vi "PushElement.vi"(8 "error in (no error)":errorcluster, 10 "open list element":T1, 11 "Astar Open List in":refnum<class "NI_Robotics_Priority Queue.lvclass">) -> (0 "error out":errorcluster, 3 "Astar Open List out":refnum<class "NI_Robotics_Priority Queue.lvclass">)   [LabVIEW 2017, in "NI_Robotics_Priority Queue.lvclass"]
uses:
  <vilib>/robotics/Navigation/shared/Priority Queue/NI_Robotics_Priority Queue.lvclass
  <vilib>/robotics/Navigation/shared/Priority Queue/Open List Element.ctl
  <vilib>/robotics/Navigation/shared/MapNode/AbstractMapNode/NI_Robotics_AbstractMapNode.lvclass
  <vilib>/robotics/Navigation/shared/Priority Queue/NI_Robotics_Priority Queue.lvclass/NI_Robotics_Priority Queue.ctl
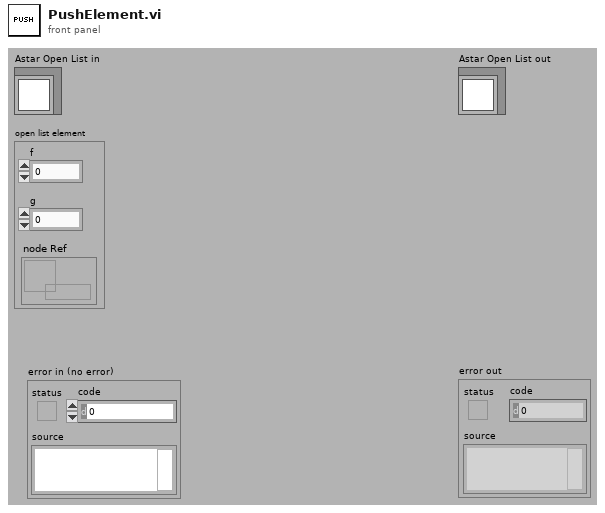
[diagram p1: front panel]
types:
  T1 = typedef "NI_Robotics_Priority Queue.lvclass/Open List Element.ctl" = cluster{"f":dbl, "g":dbl, "node Ref":refnum<data-value>}
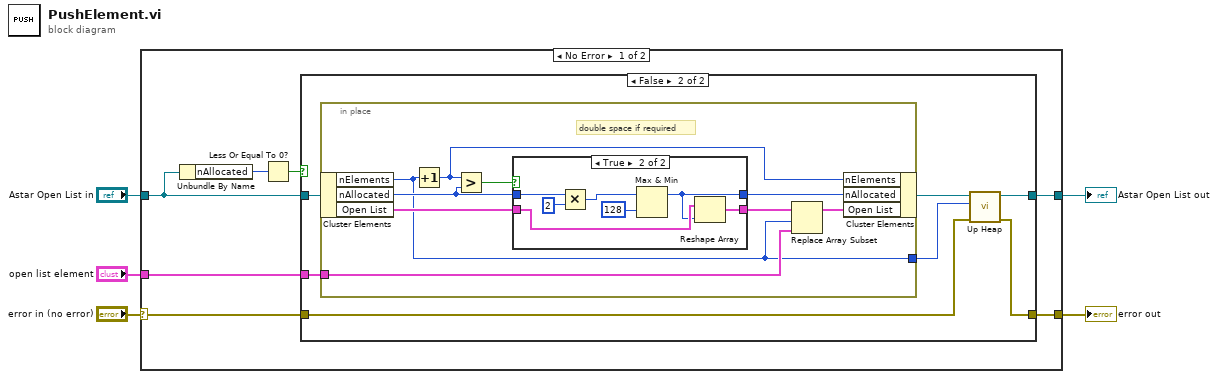
[diagram p0: block diagram]
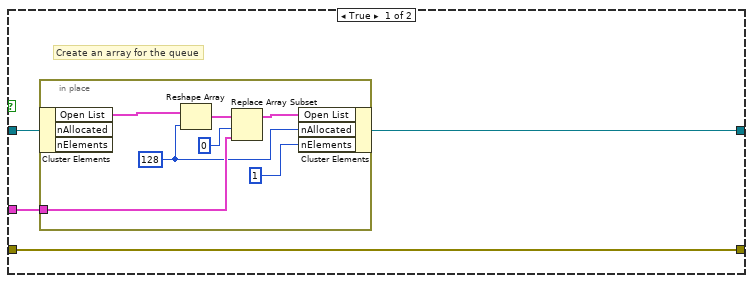
[diagram p2: hidden frame]
diagram:
  n1 = case shown="No Error" "error in (no error)" {
    selector: "error in (no error)" -> [w6 w49]
    tunnel: "Astar Open List in" -> [w12 w50]
    tunnel: "open list element" -> [w11 _]
    tunnel: [w10 w50] -> w3
    tunnel: [w9 w49] -> w2
    frame No Error {
      n2 = Unbundle By Name(w12) -> ("nAllocated"=w8:i32)
      n3 = Less Or Equal To 0?(x=w8) -> (x <= 0?=w7:bool)
      n4 = case shown="False" w7 {
        tunnel: w12 -> [w16 w30]
        tunnel: w11 -> [w15 w29]
        tunnel: [w14 w26] -> w10
        tunnel: w6 -> [w13 w25]
        tunnel: [w13 w24] -> w9
        frame True {
          # "Create an array for the queue"
          n5 = in-place {
            in-place-border: w15 -> [w20]
            w19 = 128 ("dimension size")
            n6 = in-place-cluster #1(w16) -> ("Open List"=w23:T1[])  [unwired: 2 out]
            n7 = Reshape Array(w23, w19) -> (w22:T1[])
            n8 = Replace Array Subset(array=w22, new element=w20, index=0) -> (w18:T1[])
            n9 = in-place-cluster #1("Open List"=w18, "nAllocated"=w19, "nElements"=1) -> (w14:refnum<class "NI_Robotics_Priority Queue.lvclass">)
          }
        }
        frame False {
          n10 = in-place {
            in-place-border: w29 -> [w34]
            in-place-border: [w31] -> w28
            # "double space if required"
            n11 = in-place-cluster #2(w30) -> ("nElements"=w31:i32, "nAllocated"=w38:i32, "Open List"=w37:T1[])
            n12 = Increment(x=w31) -> (x+1=w33:i32)
            n13 = Greater?(x=w33, y=w38) -> (0:w39:bool)
            n14 = case shown="True" w39 {
              tunnel: w38 -> [w41 w48]
              tunnel: w37 -> [w40 w44]
              tunnel: [w40 w43] -> w35
              tunnel: [w41 w42] -> w36
              frame False {
              }
              frame True {
                n15 = Multiply(x=w48, y=2) -> (x*y=w46:i32)
                n16 = Max & Min(x=w46, y=128) -> (max(x,y)=w42:i32)  [unwired: 1 out]
                n17 = Reshape Array(w44, w42) -> (w43:T1[])
              }
            }
            n18 = Replace Array Subset(array=w35, new element=w34, index=w31) -> (w32:T1[])
            n19 = in-place-cluster #2("nElements"=w33, "nAllocated"=w36, "Open List"=w32) -> (w27:refnum<class "NI_Robotics_Priority Queue.lvclass">)
          }
          n20 = call <vilib>:"Up Heap.vi"("error in (no error)"=w25, "index"=w28, "Astar Open List in"=w27) -> ("error out"=w24:errorcluster, "Astar Open List out"=w26:refnum<class "NI_Robotics_Priority Queue.lvclass">)  [unwired: 7 in]
        }
      }
    }
    frame Error {
    }
  }
  "error out" <- w2
  "Astar Open List out" <- w3
